vi "参数设置页.vi"() -> ()   [LabVIEW 2016, in "斯坦道CODMn.lvlib"]
uses:
  <vilib>/Utility/config.llb/NI_LVConfig.lvlib
panel:
  in  "采水泵排液时间/s:":i32
  in  "采水泵沉淀时间/s:":i32
  in  "采水泵润洗时间/s:":i32
  in  "采水泵进样时间/s:":i32
  in  "标度泵计量数 2":dbl
  in  "零点泵计量数 2":dbl
  in  "氢氧化钠:":dbl
  in  "屏蔽负值":bool
  in  "常规版/认证版":enum16{"常规版-酸性", "常规版-碱性", "认证版", "浮台版"}(ring)
  out "稀释倍数解释":string
  in  "CODMn零点核查选择":enum16{"零点核查走纯水管", "零点核查走零漂管"}(ring)
  in  "低量程稀释倍数:":dbl=1.0
  in  "高量程稀释倍数:":dbl=2.0
  in  "零点液自动补测":bool
  in  "跨度液自动补测":bool
  in  "标准液自动补测":bool
  in  "零点液偏差":dbl
  in  "跨度液偏差":dbl
  in  "标准液偏差":dbl
  in  "更换泵管":bool
  in  "跨度值":dbl
  in  "加标回收量程：":enum32{"H", "L", "AUTO"}(ring)=enum."AUTO"
  out "CODMn序列号":string
  out "CODMn软件版本：":string
  in  "标样核查量程选择":enum32{"H", "L", "AUTO"}(ring)=enum."AUTO"
  in  "标样浓度":dbl
  in  "零点核查量程选择":enum32{"H", "L", "AUTO"}(ring)=enum."AUTO"
  in  "零点核查浓度":dbl
  in  "跨度量程选择":enum32{"H", "L", "AUTO"}(ring)=enum."AUTO"
  in  "跨度液浓度":dbl
  in  "水样：":dbl
  in  "蒸馏水：":dbl
  in  "标液：":dbl
  in  "零点核查样：":dbl
  in  "加标回收样：":dbl
  in  "草酸钠":dbl
  in  "高锰酸钾":dbl
  in  "硫酸":dbl
  out "量程解释说明":string
  in  "高切低阈值:":dbl
  in  "低切高阈值:":dbl
  in  "水样量程选择:":enum16{"L", "H", "自动切换测一次", "自动切换测两次"}(ring)
  in  "标准液浓度":dbl
  in  "温度":dbl
  in  "恒温时间":dbl
  in  "当前量程：":enum16{"L", "H"}(ring)
  # "基本参数设置"
  # "泵计量参数设置"
  # "高锰酸钾："
  # "加热恒温温度(℃):"
  # "草酸钠："
  # "恒温时间(分钟):"
  # "硫酸："
  # "标准液浓度(mg/L):"
  # "跨度核查浓度："
  # "零点液偏差±:"
  # "标准液偏差%:"
  # "跨度核查量程："
  # "跨度液偏差%:"
  # "零点核查浓度："
  # "标样浓度："
  # "零点核查量程："
  # "标样核查量程："
  # "跨度值:"
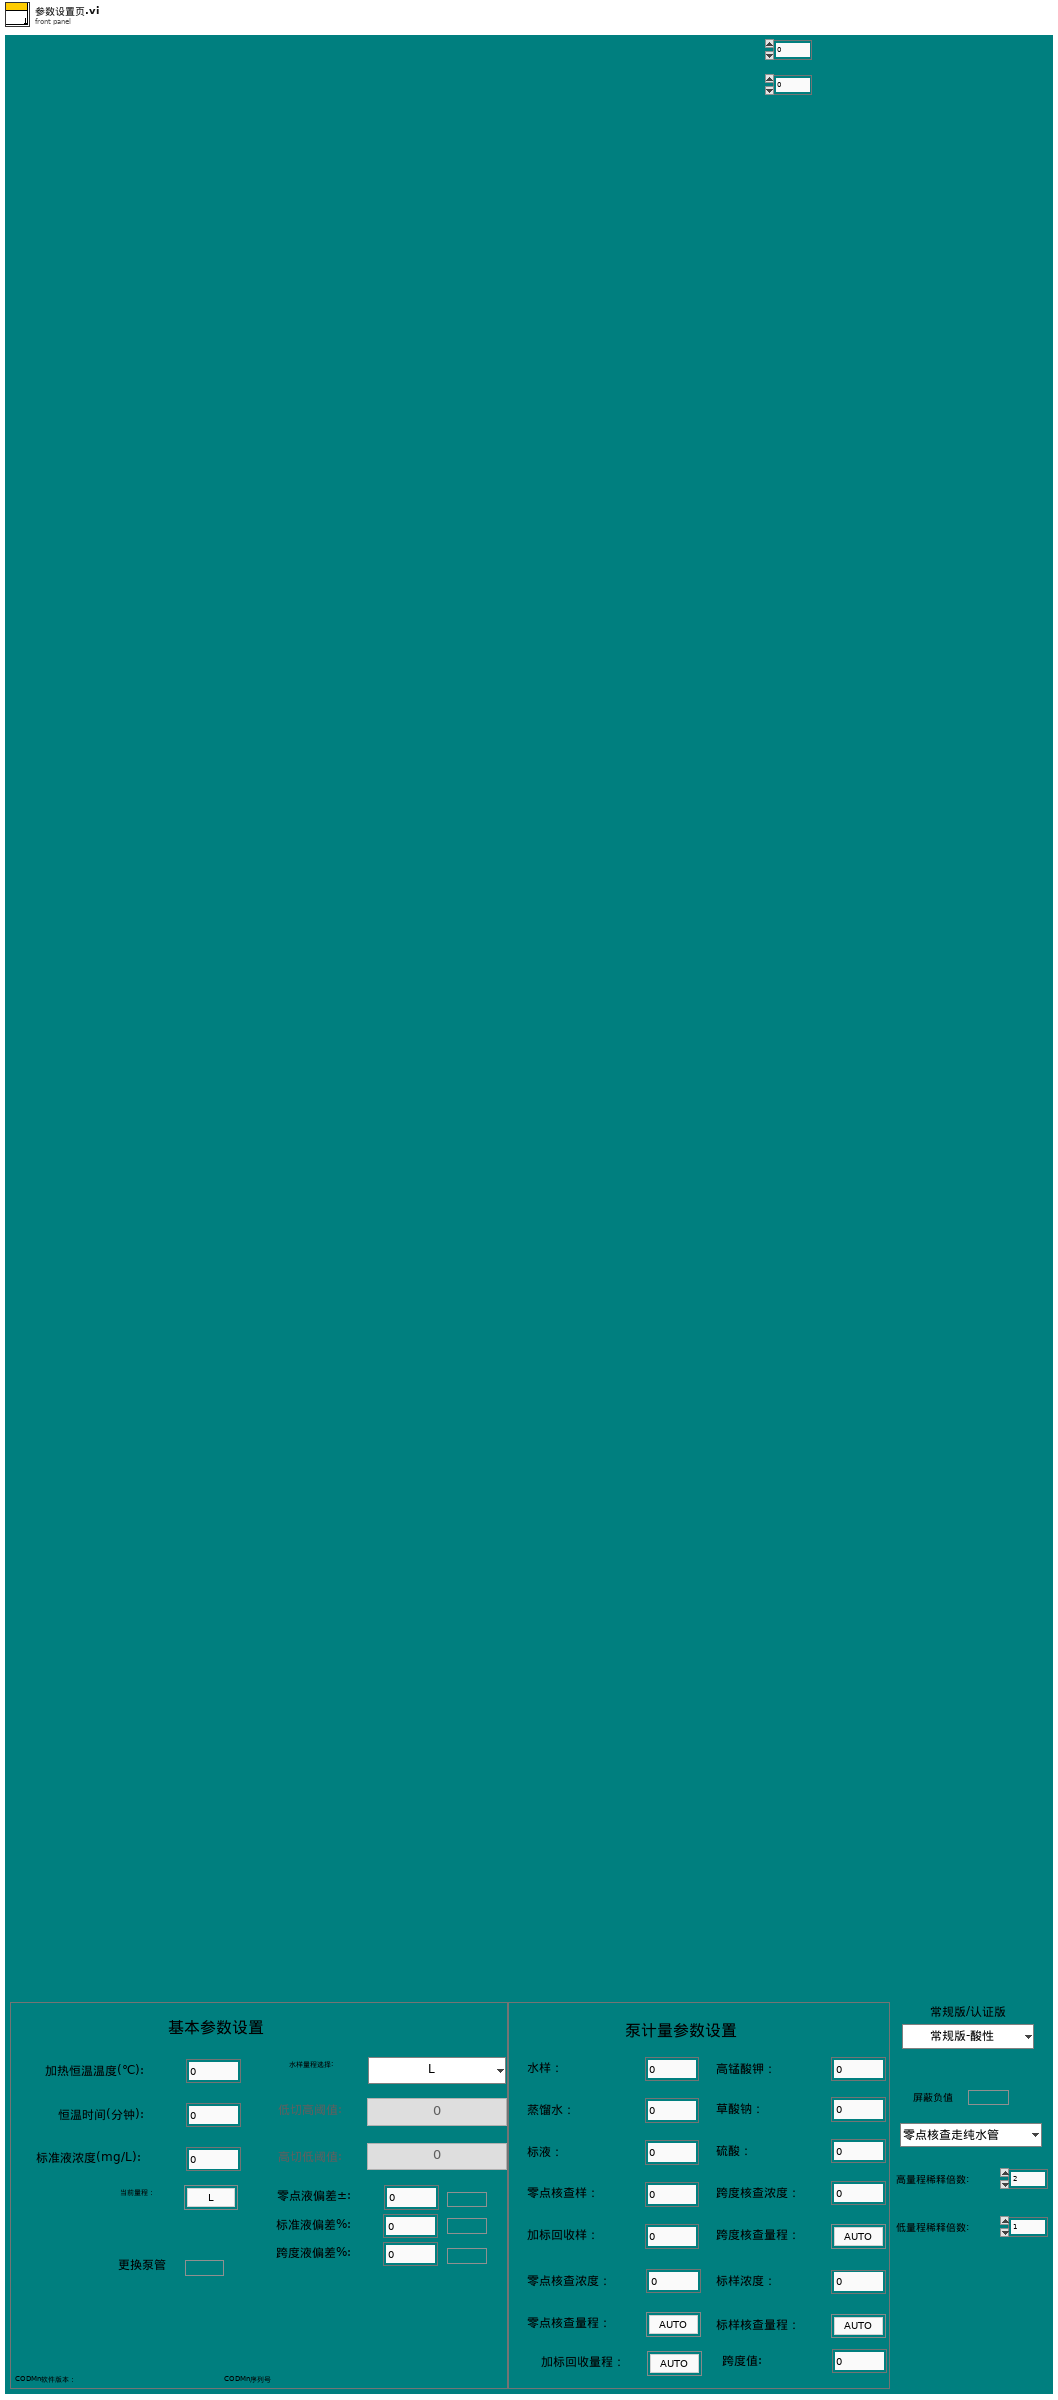
[diagram p1: front panel]
types:
  T1 = typedef "NI_LVConfig.lvlib/Config Data RefNum.ctl" = refnum<k1>
  T2 = cluster{"时间":timestamp, "水样计量数":u16, "蒸馏水计量数":u16, "标液计量数":u16, "零点核查计量数":u16, "加标回收计量数":u16, "硫酸计量数":u16, "高锰酸钾计量数":u16, "草酸钠计量数":u16, "更换泵管":string}
  T3 = cluster{"测量量程":dbl, "测量精度":dbl, "测量间隔":dbl, "消解温度":dbl, "消解时长":dbl, "空白校准时间":timestamp, "曲线截距":dbl, "曲线斜率":dbl, "测量检出限":dbl, "测量信号值":dbl, "线性相关系数":dbl, "二次多项式系数":dbl, "标样校准时间":timestamp, "稀释倍数":dbl, "三项式系数":dbl, "空白标定系数":dbl, "量程系数":dbl, "F0/ORPA":dbl, "F1/ORPB":dbl, "F2/ORPK":dbl, "F3":dbl, "F4":dbl, "F5":dbl, "F6":dbl, "F7":dbl, "X0/滴定数":dbl, "量程":dbl}
  T4 = enum8{"Enabled", "Disabled", "Disabled and Grayed Out"}
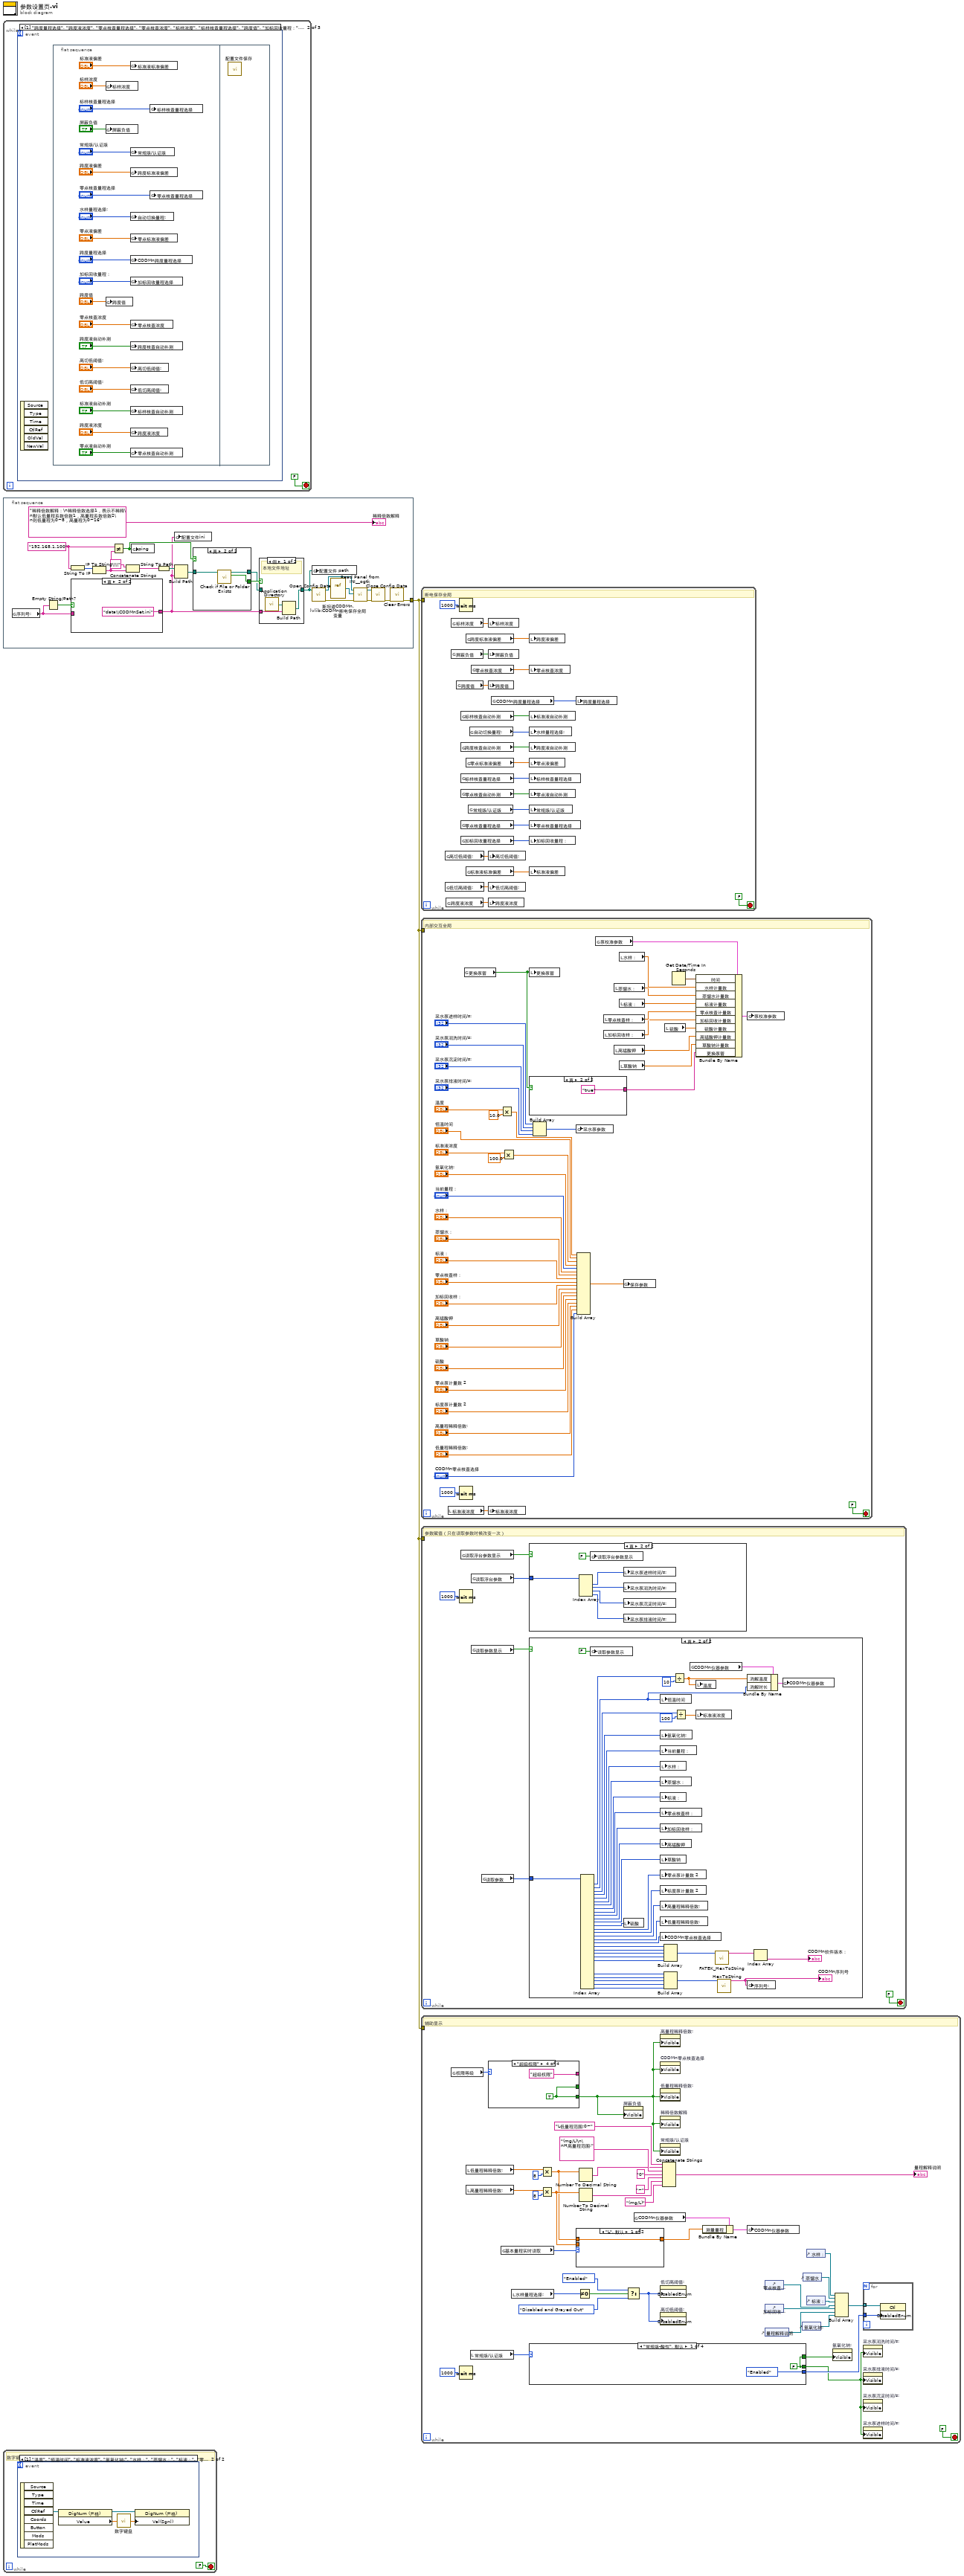
[diagram p0: block diagram]
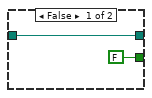
[diagram p2: hidden frame]
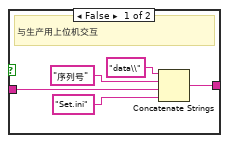
[diagram p4: hidden frame]
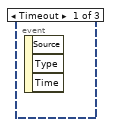
[diagram p5: hidden frame]
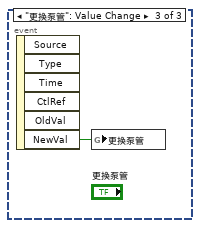
[diagram p6: hidden frame]
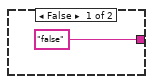
[diagram p9: hidden frame]
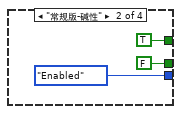
[diagram p10: hidden frame]
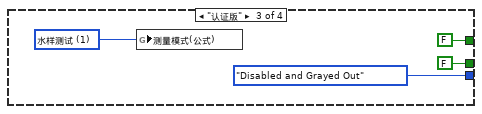
[diagram p11: hidden frame]
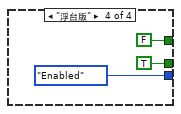
[diagram p12: hidden frame]
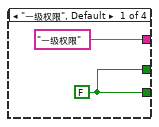
[diagram p13: hidden frame]
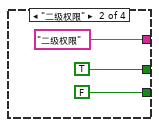
[diagram p14: hidden frame]
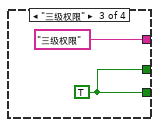
[diagram p15: hidden frame]
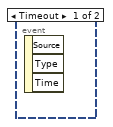
[diagram p17: hidden frame]
diagram:
  n1 = while {
    stop <- FALSE stop-if-true
    n2 = event shown="[1] \"跨度量程选择\", \"跨度液浓度\", \"零点核查量程选择\", \"零点核查浓度\", \"标样浓度\", \"标样核查量程选择\", \"跨度值\", \"加标回收量程：\", \"标准液偏差\", \"跨度液偏差\", \"零点液偏差\", \"标准液自动补测\", \"跨度液自动补测\", \"零点液自动补测\", \"常规版/认证版\", \"屏蔽负值\", \"水样量程选择:\", \"低切高阈值:\", \"高切低阈值:\": 值改变" {
      selector: _ -> [_ _ _]
      dyn-events: _ -> [_ _ _]
      timeout: _ -> [_ _ _]
      event Timeout {
        n3 = event-data() -> ()  [unwired: 1 in, 3 out]
      }
      event "跨度量程选择", "跨度液浓度", "零点核查量程选择", "零点核查浓度", "标样浓度", "标样核查量程选择", "跨度值", "加标回收量程：", "标准液偏差", "跨度液偏差", "零点液偏差", "标准液自动补测", "跨度液自动补测", "零点液自动补测", "常规版/认证版", "屏蔽负值", "水样量程选择:", "低切高阈值:", "高切低阈值:": Value Change {
        n4 = event-data() -> ()  [unwired: 1 in, 6 out]
        n5 = flat-sequence {
          frame #0 {
            n6 = global write "CODMn断电保存全局变量.vi" "标样浓度"("标样浓度") -> ()
            n7 = global write "CODMn断电保存全局变量.vi" "屏蔽负值"("屏蔽负值") -> ()
            n8 = global write "CODMn断电保存全局变量.vi" "跨度值"("跨度值") -> ()
            n9 = global write "CODMn断电保存全局变量.vi" "标准液标准偏差"("标准液偏差") -> ()
            n10 = global write "CODMn断电保存全局变量.vi" "常规版/认证版"("常规版/认证版") -> ()
            n11 = global write "CODMn断电保存全局变量.vi" "跨度标准液偏差"("跨度液偏差") -> ()
            n12 = global write "CODMn断电保存全局变量.vi" "自动切换量程:"("水样量程选择:") -> ()
            n13 = global write "CODMn断电保存全局变量.vi" "零点标准液偏差"("零点液偏差") -> ()
            n14 = global write "CODMn断电保存全局变量.vi" "CODMn跨度量程选择"("跨度量程选择") -> ()
            n15 = global write "CODMn断电保存全局变量.vi" "加标回收量程选择"("加标回收量程：") -> ()
            n16 = global write "CODMn断电保存全局变量.vi" "零点核查浓度"("零点核查浓度") -> ()
            n17 = global write "CODMn断电保存全局变量.vi" "跨度核查自动补测"("跨度液自动补测") -> ()
            n18 = global write "CODMn断电保存全局变量.vi" "高切低阈值:"("高切低阈值:") -> ()
            n19 = global write "CODMn断电保存全局变量.vi" "低切高阈值:"("低切高阈值:") -> ()
            n20 = global write "CODMn断电保存全局变量.vi" "标样核查自动补测"("标准液自动补测") -> ()
            n21 = global write "CODMn断电保存全局变量.vi" "跨度液浓度"("跨度液浓度") -> ()
            n22 = global write "CODMn断电保存全局变量.vi" "零点核查自动补测"("零点液自动补测") -> ()
            n23 = global write "CODMn断电保存全局变量.vi" "标样核查量程选择"("标样核查量程选择") -> ()
            n24 = global write "CODMn断电保存全局变量.vi" "零点核查量程选择"("零点核查量程选择") -> ()
          }
          frame #1 {
            n25 = call "配置文件保存.vi"() -> ()  [unwired: 12 in]
          }
        }
      }
      event "更换泵管": Value Change {
        n26 = event-data() -> ("NewVal"=w22:bool)  [unwired: 1 in, 5 out]
        n27 = global write "COD内部交互全局.vi" "更换泵管"(w22) -> ()
      }
    }
  }
  n28 = flat-sequence {
    tunnel: [w23] -> w1
    frame #0 {
      w39 = "192.168.1.100" ("名称")
      n29 = global read "COD内部交互全局.vi" "序列号:"() -> (w43:string)
      n30 = Empty String/Path?(string/path=w43) -> (empty?=w24:bool)
      n31 = String To IP(1:w39) -> (0:w32:u32)
      n32 = case shown="真" w24 {
        tunnel: w43 -> [w55 _]
        tunnel: [w54 "data\\CODMnSet.ini" ("名称或相对路径")] -> w27
        frame False {
          # "与生产用上位机交互"
          n33 = Concatenate Strings("data\\" ("字符串"), "序列号" ("字符串"), w55, "Set.ini" ("名称或相对路径")) -> (w54:string)
        }
        frame True {
        }
      }
      n34 = IP To String(2:w32) -> (0:w35:string)  [unwired: 1 in]
      n35 = Not Equal?(x=w39, y=w35) -> (x != y?=w40:bool)
      n36 = Concatenate Strings("\\\\" ("字符串"), w35) -> (w34:string)
      n37 = global write "CODMN外部API.vi" "ping"(w40) -> ()
      n38 = String To Path(string=w34) -> (path=w41:path)
      n39 = global write "COD内部交互全局.vi" "配置文件ini"(w27) -> ()
      n40 = Build Path(base path=w41, name or relative path=w27) -> (appended path=w36:path)
      n41 = case shown="真" w40 {
        tunnel: w36 -> [w45 w49]
        tunnel: [w45 w48] -> w37
        tunnel: [FALSE w47] -> w38
        frame False {
        }
        frame True {
          n42 = call <vilib>:"Check if File or Folder Exists.vi"("path"=w49) -> ("file or folder exists?"=w47:bool, "dup path"=w48:path)  [unwired: 8 in, 1 out]
        }
      }
      n43 = case shown="假" w38 {
        tunnel: w37 -> [_ w53]
        tunnel: [w51 w53] -> w26
        tunnel: w27 -> [w50 _]
        frame False {
          # "本地文件地址"
          n44 = call <vilib>:"Application Directory.vi"() -> ("Application Directory"=w52:path)
          n45 = Build Path(base path=w52, name or relative path=w50) -> (appended path=w51:path)
        }
        frame True {
          # "网络共享地址"
        }
      }
      n46 = global write "CODMN外部API.vi" "配置文件 path"(w26) -> ()
      n47 = call <vilib>:"Open Config Data.vi"("configuration file path"=w26) -> ("error out"=w28:errorcluster, "refnum"=w29:T1)  [unwired: 8 in, 1 out]
      n48 = vi-ref "斯坦道CODMn.lvlib:CODMn断电保存全局变量.vi"() -> (w42:refnum<vi>)
      n49 = call <userlib>:"Read Panel from INI__ogtk.vi"("error in (no error)"=w28, "VI ref"=w42, "refnum"=w29) -> ("error out"=w30:errorcluster, "refnum out"=w31:T1)  [unwired: 7 in]
      n50 = call <vilib>:"Close Config Data.vi"("error in (no error)"=w30, "refnum"=w31) -> ("error out"=w25:errorcluster)  [unwired: 8 in, 1 out]
      n51 = call <vilib>:"Clear Errors.vi"("error in (no error)"=w25) -> ("error out"=w23:errorcluster)  [unwired: 5 in, 1 out]
      "稀释倍数解释" <- "稀释倍数解释：\n稀释倍数选择1，表示不稀释\n默认低量程系数倍数1，高量程系数倍数2\n则低量程为0~8，高量程为0~16" ("稀释倍数解释")
    }
  }
  n52 = while {
    stop <- FALSE stop-if-true
    # "数字键盘输入"
    n53 = event shown="[1] \"温度\", \"恒温时间\", \"标准液浓度\", \"氢氧化钠:\", \"水样：\", \"蒸馏水：\", \"标液：\", \"零点核查样：\", \"加标回收样：\", \"草酸钠\", \"高锰酸钾\", \"硫酸\", \"高量程稀释倍数:\", \"低量程稀释倍数:\", \"跨度液浓度\", \"零点核查浓度\", \"标样浓度\", \"标准液偏差\", \"跨度液偏差\", \"零点液偏差\", \"低切高阈值:\", \"高切低阈值:\": 鼠标按下" {
      selector: _ -> [_ _]
      dyn-events: _ -> [_ _]
      timeout: _ -> [_ _]
      event Timeout {
        n54 = event-data() -> ()  [unwired: 1 in, 3 out]
      }
      event "温度", "恒温时间", "标准液浓度", "氢氧化钠:", "水样：", "蒸馏水：", "标液：", "零点核查样：", "加标回收样：", "草酸钠", "高锰酸钾", "硫酸", "高量程稀释倍数:", "低量程稀释倍数:", "跨度液浓度", "零点核查浓度", "标样浓度", "标准液偏差", "跨度液偏差", "零点液偏差", "低切高阈值:", "高切低阈值:": Mouse Down {
        n55 = event-data() -> ("CtlRef"=w64:refnum<vi>)  [unwired: 1 in, 7 out]
        n56 = property class="DigNum (严格)"(reference=w64) -> (reference out=w62:refnum<vi>, "Value"=w63:dbl)  [unwired: 1 in, 1 out]
        n57 = call "数字键盘.vi"("OldNumber"=w63) -> ("NewNumber"=w61:sgl)
        n58 = property class="DigNum (严格)"(reference=w62, "Val(Sgnl)"=w61) -> ()  [unwired: 1 in, 2 out]
      }
    }
  }
  n59 = while {
    tunnel: w1 -> [_]
    stop <- FALSE stop-if-true
    # "断电保存全局"
    n60 = global read "CODMn断电保存全局变量.vi" "高切低阈值:"() -> (w82:dbl)
    n61 = global read "CODMn断电保存全局变量.vi" "低切高阈值:"() -> (w83:dbl)
    n62 = global read "CODMn断电保存全局变量.vi" "跨度液浓度"() -> (w66:dbl)
    n63 = global read "CODMn断电保存全局变量.vi" "标样浓度"() -> (w65:dbl)
    n64 = global read "CODMn断电保存全局变量.vi" "屏蔽负值"() -> (w77:bool)
    n65 = global read "CODMn断电保存全局变量.vi" "跨度值"() -> (w67:dbl)
    n66 = Wait (ms)(milliseconds to wait=u32 1000 ("等待时间（毫秒）")) -> ()  [unwired: 1 out]
    n67 = global read "CODMn断电保存全局变量.vi" "标样核查自动补测"() -> (w75:bool)
    n68 = global read "CODMn断电保存全局变量.vi" "跨度核查自动补测"() -> (w74:bool)
    n69 = global read "CODMn断电保存全局变量.vi" "标样核查量程选择"() -> (w80:enum32{"H", "L", "AUTO"})
    n70 = global read "CODMn断电保存全局变量.vi" "零点核查自动补测"() -> (w76:bool)
    n71 = global read "CODMn断电保存全局变量.vi" "零点核查量程选择"() -> (w70:enum32{"H", "L", "AUTO"})
    n72 = global read "CODMn断电保存全局变量.vi" "加标回收量程选择"() -> (w69:enum32{"H", "L", "AUTO"})
    n73 = global read "CODMn断电保存全局变量.vi" "跨度标准液偏差"() -> (w71:dbl)
    n74 = global read "CODMn断电保存全局变量.vi" "零点标准液偏差"() -> (w72:dbl)
    n75 = global read "CODMn断电保存全局变量.vi" "标准液标准偏差"() -> (w73:dbl)
    n76 = global read "CODMn断电保存全局变量.vi" "常规版/认证版"() -> (w78:enum16{"常规版-酸性", "常规版-碱性", "认证版", "浮台版"})
    n77 = global read "CODMn断电保存全局变量.vi" "自动切换量程:"() -> (w81:enum16{"L", "H", "自动切换测一次", "自动切换测两次"})
    n78 = global read "CODMn断电保存全局变量.vi" "零点核查浓度"() -> (w68:dbl)
    n79 = local write "标样浓度"(w65) -> ()
    n80 = local write "屏蔽负值"(w77) -> ()
    n81 = local write "跨度值"(w67) -> ()
    n82 = local write "高切低阈值:"(w82) -> ()
    n83 = local write "低切高阈值:"(w83) -> ()
    n84 = local write "跨度液浓度"(w66) -> ()
    n85 = global read "CODMn断电保存全局变量.vi" "CODMn跨度量程选择"() -> (w79:enum32{"H", "L", "AUTO"})
    n86 = local write "跨度液偏差"(w71) -> ()
    n87 = local write "零点核查浓度"(w68) -> ()
    n88 = local write "标准液自动补测"(w75) -> ()
    n89 = local write "水样量程选择:"(w81) -> ()
    n90 = local write "跨度液自动补测"(w74) -> ()
    n91 = local write "零点液偏差"(w72) -> ()
    n92 = local write "标样核查量程选择"(w80) -> ()
    n93 = local write "零点液自动补测"(w76) -> ()
    n94 = local write "常规版/认证版"(w78) -> ()
    n95 = local write "零点核查量程选择"(w70) -> ()
    n96 = local write "加标回收量程："(w69) -> ()
    n97 = local write "标准液偏差"(w73) -> ()
    n98 = local write "跨度量程选择"(w79) -> ()
  }
  n99 = while {
    tunnel: w1 -> [_]
    stop <- FALSE stop-if-true
    # "内部交互全局"
    n100 = local read "标准液浓度"() -> (w127:dbl)
    n101 = Wait (ms)(milliseconds to wait=u32 1000 ("等待时间（毫秒）")) -> ()  [unwired: 1 out]
    n102 = global read "COD内部交互全局.vi" "更换泵管"() -> (w86:bool)
    n103 = global write "COD浓度全局变量.vi" "标准液浓度"(w127) -> ()
    n104 = Multiply(x="温度", y=10.0) -> (x*y=w107:dbl)
    n105 = Multiply(x="标准液浓度", y=100.0) -> (x*y=w109:dbl)
    n106 = local write "更换泵管"(w86) -> ()
    n107 = case shown="真" w86 {
      tunnel: ["false" "true"] -> w95
      frame False {
      }
      frame True {
      }
    }
    n108 = Build Array("采水泵进样时间/s:", "采水泵润洗时间/s:", "采水泵沉淀时间/s:", "采水泵排液时间/s:") -> (w103:i32[])
    n109 = global write "COD内部交互全局.vi" "采水泵参数"(w103) -> ()
    n110 = Build Array(w107, "恒温时间", w109, "氢氧化钠:", "当前量程：", "水样：", "蒸馏水：", "标液：", "零点核查样：", "加标回收样：", "高锰酸钾", "草酸钠", "硫酸", "零点泵计量数 2", "标度泵计量数 2", "高量程稀释倍数:", "低量程稀释倍数:", "CODMn零点核查选择") -> (w110:dbl[])
    n111 = global read "COD内部交互全局.vi" "泵校准参数"() -> (w98:T2)
    n112 = local read "零点核查样："() -> (w91:dbl)
    n113 = local read "加标回收样："() -> (w90:dbl)
    n114 = local read "蒸馏水："() -> (w93:dbl)
    n115 = local read "高锰酸钾"() -> (w88:dbl)
    n116 = local read "水样："() -> (w94:dbl)
    n117 = local read "标液："() -> (w92:dbl)
    n118 = local read "草酸钠"() -> (w87:dbl)
    n119 = global write "COD内部交互全局.vi" "保存参数"(w110) -> ()
    n120 = local read "硫酸"() -> (w89:dbl)
    n121 = Get Date/Time In Seconds() -> (seconds since 1Jan1904=w96:timestamp)
    n122 = Bundle By Name(cluster=w98, "时间"=w96, "水样计量数"=w94, "蒸馏水计量数"=w93, "标液计量数"=w92, "零点核查计量数"=w91, "加标回收计量数"=w90, "硫酸计量数"=w89, "高锰酸钾计量数"=w88, "草酸钠计量数"=w87, "更换泵管"=w95) -> (w97:T2)
    n123 = global write "COD内部交互全局.vi" "泵校准参数"(w97) -> ()
  }
  n124 = while {
    tunnel: w1 -> [_]
    stop <- FALSE stop-if-true
    # "参数赋值（只在读取参数时候改变一次）"
    n125 = Wait (ms)(milliseconds to wait=u32 1000 ("等待时间（毫秒）")) -> ()  [unwired: 1 out]
    n126 = global read "COD内部交互全局.vi" "读取浮台参数显示"() -> (w136:bool)
    n127 = global read "COD内部交互全局.vi" "读取浮台参数"() -> (w135:u16[])
    n128 = global read "COD内部交互全局.vi" "读取参数显示"() -> (w133:bool)
    n129 = global read "COD内部交互全局.vi" "读取参数"() -> (w132:u16[])
    n130 = case shown="真" w136 {
      tunnel: w135 -> [_ w183]
      frame False {
      }
      frame True {
        n131 = Index Array(array=w183) -> (element #1=w182:u16, element #2=w181:u16, element #3=w180:u16, element #4=w179:u16)  [unwired: 4 in]
        n132 = global write "COD内部交互全局.vi" "读取浮台参数显示"(FALSE ("读取参数显示")) -> ()
        n133 = local write "采水泵进样时间/s:"(w182) -> ()
        n134 = local write "采水泵润洗时间/s:"(w181) -> ()
        n135 = local write "采水泵沉淀时间/s:"(w180) -> ()
        n136 = local write "采水泵排液时间/s:"(w179) -> ()
      }
    }
    n137 = case shown="真" w133 {
      tunnel: w132 -> [_ w177]
      frame False {
      }
      frame True {
        n138 = Index Array(array=w177) -> (element #1=w175:u16, element #2=w171:u16, element #3=w169:u16, element #4=w167:u16, element #5=w166:u16, element #6=w165:u16, element #7=w164:u16, element #8=w163:u16, element #9=w162:u16, element #10=w161:u16, element #11=w160:u16, element #12=w159:u16, element #13=w158:u16, element #14=w157:u16, element #15=w156:u16, element #16=w155:u16, element #17=w154:u16, element #18=w148:u16, element #19=w147:u16, element #20=w146:u16, element #21=w145:u16, element #22=w144:u16, element #23=w143:u16, element #27=w142:u16, element #28=w141:u16, element #29=w140:u16, element #30=w139:u16, element #31=w138:u16)  [unwired: 31 in, 3 out]
        n139 = global write "COD内部交互全局.vi" "读取参数显示"(FALSE ("读取参数显示")) -> ()
        n140 = local write "硫酸"(w158) -> ()
        n141 = local write "恒温时间"(w171) -> ()
        n142 = local write "氢氧化钠:"(w167) -> ()
        n143 = local write "当前量程："(w166) -> ()
        n144 = local write "水样："(w165) -> ()
        n145 = local write "蒸馏水："(w164) -> ()
        n146 = local write "标液："(w163) -> ()
        n147 = local write "零点核查样："(w162) -> ()
        n148 = local write "加标回收样："(w161) -> ()
        n149 = local write "高锰酸钾"(w160) -> ()
        n150 = local write "草酸钠"(w159) -> ()
        n151 = local write "零点泵计量数 2"(w157) -> ()
        n152 = local write "标度泵计量数 2"(w156) -> ()
        n153 = local write "高量程稀释倍数:"(w155) -> ()
        n154 = local write "低量程稀释倍数:"(w154) -> ()
        n155 = local write "CODMn零点核查选择"(w148) -> ()
        n156 = Build Array(w147, w146, w145, w144, w143) -> (w153:u16[])
        n157 = Build Array(w142, w141, w140, w139, w138) -> (w152:u16[])
        n158 = Divide(x=w175, y=u16 10) -> (x/y=w172:dbl)
        n159 = Divide(x=w169, y=u16 100) -> (x/y=w168:dbl)
        n160 = global read "CODMn断电保存全局变量.vi" "CODMn仪器参数"() -> (w174:T3)
        n161 = local write "温度"(w172) -> ()
        n162 = local write "标准液浓度"(w168) -> ()
        n163 = call "FATEK_HexToString.vi"("数组"=w153) -> ("STRING"=w151:string[])  [unwired: 10 in]
        n164 = call "HexToString.vi"("数组"=w152) -> ("字符串"=w149:string)  [unwired: 10 in]
        "CODMn序列号" <- w149
        n165 = Bundle By Name(cluster=w174, "消解温度"=w172, "消解时长"=w171) -> (w173:T3)
        n166 = global write "COD内部交互全局.vi" "序列号:"(w149) -> ()
        n167 = Index Array(array=w151) -> (element=→"CODMn软件版本：":string)  [unwired: 1 in]
        n168 = global write "CODMn断电保存全局变量.vi" "CODMn仪器参数"(w173) -> ()
      }
    }
  }
  n169 = while {
    tunnel: w1 -> [_]
    stop <- FALSE stop-if-true
    # "辅助显示"
    n170 = global read "CODMN外部API.vi" "权限等级"() -> (w203:enum16{"一级权限", "二级权限", "三级权限", "超级权限"})
    n171 = Wait (ms)(milliseconds to wait=u32 1000 ("等待时间（毫秒）")) -> ()  [unwired: 1 out]
    n172 = local read "低量程稀释倍数:"() -> (w219:dbl)
    n173 = local read "高量程稀释倍数:"() -> (w211:dbl)
    n174 = local read "常规版/认证版"() -> (w193:enum16{"常规版-酸性", "常规版-碱性", "认证版", "浮台版"})
    n175 = case shown="\"超级权限\"" w203 {
      tunnel: [w238 FALSE w243 w245] -> w202
      tunnel: ["一级权限" "二级权限" "三级权限" "超级权限"] -> _
      tunnel: [w238 TRUE w243 w245] -> _
      frame "一级权限", Default {
        w238 = FALSE
      }
      frame "二级权限" {
      }
      frame "三级权限" {
        w243 = TRUE
      }
      frame "超级权限" {
        w245 = TRUE
      }
    }
    n176 = global read "COD内部交互全局.vi" "基本量程实时读取"() -> (w207:enum16{"L", "H", "AUTO"})
    n177 = local read "水样量程选择:"() -> (w186:enum16{"L", "H", "自动切换测一次", "自动切换测两次"})
    n178 = case shown="\"常规版-酸性\", 默认" w193 {
      tunnel: [T4."Enabled" ("禁用") T4."Enabled" ("禁用") T4."Disabled and Grayed Out" ("禁用") T4."Enabled" ("禁用")] -> w192
      tunnel: [w224 TRUE FALSE FALSE] -> w191
      tunnel: [w224 FALSE FALSE TRUE] -> w190
      frame "常规版-酸性", Default {
        w224 = FALSE
      }
      frame "常规版-碱性" {
      }
      frame "认证版" {
        w231 = u16 1 items=["水样测试"=1, "标样核查"=2, "零点核查"=3, "跨度核查"=4, "空白测试"=5, "平行样"=6, "加标回收"=7] ("测量模式(公式)")
        n179 = global write "CODMn断电保存全局变量.vi" "测量模式(公式)"(w231) -> ()
      }
      frame "浮台版" {
      }
    }
    n180 = Multiply(x=w219, y=i8 8) -> (x*y=w205:dbl)
    n181 = Multiply(x=w211, y=i8 8) -> (x*y=w206:dbl)
    n182 = case shown="\"L\", 默认" w207 {
      tunnel: w206 -> [_ w248]
      tunnel: [w247 w248] -> w204
      tunnel: w205 -> [w247 _]
      frame "L", Default {
      }
      frame "H" {
      }
    }
    n183 = Not Equal To 0?(x=w186) -> (x != 0?=w187:bool)
    n184 = Number To Decimal String(number=w205) -> (decimal integer string=w216:string)  [unwired: 1 in]
    n185 = Number To Decimal String(number=w206) -> (decimal integer string=w214:string)  [unwired: 1 in]
    n186 = property on="屏蔽负值" class="Bool (严格)"("Visible"=w202) -> ()  [unwired: 2 in, 2 out]
    n187 = Select(t=T4."Enabled" ("禁用"), s=w187, f=T4."Disabled and Grayed Out" ("禁用")) -> (s? t:f=w185:T4)
    n188 = global read "CODMn断电保存全局变量.vi" "CODMn仪器参数"() -> (w209:T3)
    n189 = property on="高量程稀释倍数:" class="DigNum (严格)"("Visible"=w202) -> ()  [unwired: 2 in, 2 out]
    n190 = property on="CODMn零点核查选择" class="Enum (严格)"("Visible"=w202) -> ()  [unwired: 2 in, 2 out]
    n191 = property on="低量程稀释倍数:" class="DigNum (严格)"("Visible"=w202) -> ()  [unwired: 2 in, 2 out]
    n192 = property on="稀释倍数解释" class="Str"("Visible"=w202) -> ()  [unwired: 2 in, 2 out]
    n193 = property on="常规版/认证版" class="Enum (严格)"("Visible"=w202) -> ()  [unwired: 2 in, 2 out]
    n194 = property on="低切高阈值:" class="DigNum (严格)"("DisabledEnum"=w185) -> ()  [unwired: 2 in, 2 out]
    n195 = property on="高切低阈值:" class="DigNum (严格)"("DisabledEnum"=w185) -> ()  [unwired: 2 in, 2 out]
    n196 = Concatenate Strings("L低量程范围:0~" ("量程解释说明"), w216, "(mg/L)\n\nH高量程范围:" ("量程解释说明"), "0" ("字符串"), "~" ("量程解释说明"), w214, "(mg/L)" ("量程解释说明")) -> (→"量程解释说明":string)
    n197 = Bundle By Name(cluster=w209, "测量量程"=w204) -> (w208:T3)
    n198 = global write "CODMn断电保存全局变量.vi" "CODMn仪器参数"(w208) -> ()
    n199 = control-ref of="零点核查样："() -> (w198:refnum<vi>)
    n200 = control-ref of="加标回收样："() -> (w197:refnum<vi>)
    n201 = control-ref of="量程解释说明"() -> (w196:refnum<vi>)
    n202 = control-ref of="氢氧化钠:"() -> (w195:refnum<vi>)
    n203 = control-ref of="蒸馏水："() -> (w200:refnum<vi>)
    n204 = control-ref of="水样："() -> (w201:refnum<vi>)
    n205 = control-ref of="标液："() -> (w199:refnum<vi>)
    n206 = property on="氢氧化钠:" class="DigNum (严格)"("Visible"=w191) -> ()  [unwired: 2 in, 2 out]
    n207 = Build Array(w201, w200, w199, w198, w197, w196, w195) -> (w194:refnum<vi>[])
    n208 = for {
      tunnel: w194 -> [w237] mode=indexing
      tunnel: w192 -> [w236]
      n209 = property class="Ctl"(reference=w237, "DisabledEnum"=w236) -> ()  [unwired: 1 in, 2 out]
    }
    n210 = property on="采水泵润洗时间/s:" class="DigNum (严格)"("Visible"=w190) -> ()  [unwired: 2 in, 2 out]
    n211 = property on="采水泵排液时间/s:" class="DigNum (严格)"("Visible"=w190) -> ()  [unwired: 2 in, 2 out]
    n212 = property on="采水泵沉淀时间/s:" class="DigNum (严格)"("Visible"=w190) -> ()  [unwired: 2 in, 2 out]
    n213 = property on="采水泵进样时间/s:" class="DigNum (严格)"("Visible"=w190) -> ()  [unwired: 2 in, 2 out]
  }
